vi "ble_hex2string.vi"(7 "colon?(false)":bool, 11 "Byte Array IN (index0 LS byte)":u8[](array[numeric]) format="%02x") -> (3 "HEX string OUT":string)   [LabVIEW 2017]
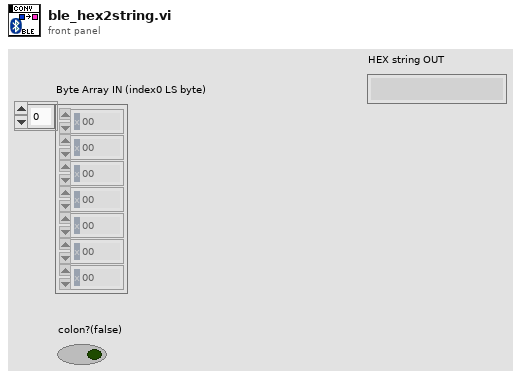
[diagram p1: front panel]
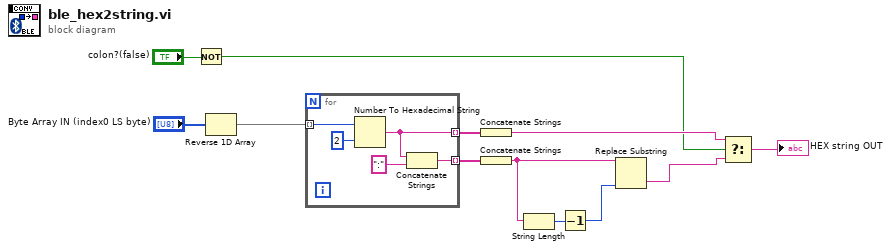
[diagram p0: block diagram]
diagram:
  n1 = Not(x="colon?(false)") -> (.not. x?=w1:bool)
  n2 = Reverse 1D Array(array="Byte Array IN (index0 LS byte)") -> (reversed array=w11:u8[])
  n3 = for {
    tunnel: w11 -> [w17] mode=indexing
    tunnel: [w15] -> w10 mode=indexing
    tunnel: [w13] -> w9 mode=indexing
    n4 = Number To Hexadecimal String(1:i16 2 ("width (-)"), 2:w17) -> (0:w15:string)
    n5 = Concatenate Strings(w15, ":") -> (w13:string)
  }
  n6 = Concatenate Strings(w10) -> (w4:string)
  n7 = Concatenate Strings(w9) -> (w8:string)
  n8 = String Length(string=w8) -> (length=w7:i32)
  n9 = Decrement(x=w7) -> (x-1=w6:i32)
  n10 = Replace Substring(2:w6, 5:w8) -> (0:w5:string)  [unwired: 2 in, 1 out]
  n11 = Select(t=w4, s=w1, f=w5) -> (s? t:f=→"HEX string OUT":string)
